vi "Autonomous Independent.vi"() -> ()   [LabVIEW 2019]
doc: "This VI is called when autonomous begins, and will automatically be terminated when autonomous ends. You can carry out timed or sensor driven robot movement independently without needing to return to the caller."
uses:
  <vilib>/Rock Robotics/Network Tables/NT Read String.vi
  Refnums.vi
  <vilib>/Rock Robotics/WPI/ThirdParty/Phoenix-LabVIEW/Motor Controller/Get/CTRE_Phoenix_MotorController_GetQuadratureData.vi
  <vilib>/addons/control/pid/pid.llb/PID (DBL).vi
  <vilib>/Rock Robotics/WPI/RobotDrive/WPI_RobotDriveArcadeDrive_Standard(NoSaturation).vi
  <vilib>/addons/control/pid/NI_PID_pid.lvlib
  <vilib>/Rock Robotics/WPI/ThirdParty/Phoenix-LabVIEW/Motor Controller/Controls/CTRE_Phoenix_MotorControl_ControlMode.ctl
panel:
  in  "Autonomous Step":T1(array[cluster]) {"Speed" min=0.0 max=1.0 step=0.01}
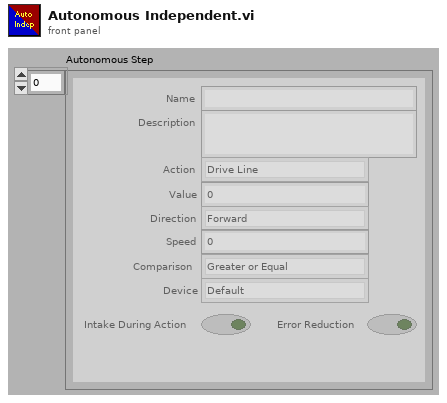
[diagram p1: front panel]
types:
  T1 = cluster{"Name":string, "Description":string, "Action":enum16{"Drive Line", "Drive Turn", "Drive Stop", "Drive Wait", "Shoot", ""}, "Value":dbl, "Direction":enum16{"Forward", "Reverse", "Left", "Right"}, "Speed":dbl, "Comparison":enum16{"Greater or Equal", "Less or Equal", "No compare (fixed)"}, "Device":enum16{"Default", "Gyro", "Laser", "Lidar", "Lime Light", "Encoder"}, "Intake During Action":bool, "Error Reduction":bool}[]
  T2 = typedef "WPI_RobotDriveDevRef.ctl" = cluster{"DevStatus":errorcluster, "Motors[]":T3[], "Square Inputs":bool, "Max Output":dbl}
  T3 = typedef "WPI_MotorControlDeviceRef.ctl" = cluster{"DeviceStatus":errorcluster, "Type":T4, "PWM":cluster{"PWM Channel":T5, "DeadBand":T6}, "CAN":cluster{"Device Number":u8, "SetOutput VI Ref":variant, "GetOutput VI Ref":variant, "Enable VI Ref":variant, "Disable VI Ref":variant, "Data":variant}, "Invert":bool, "DIO PWM":cluster{"PWM \"Enable\" Channel":T5, "DIOChannel":T7, "PWM Rate":dbl}}
  T4 = typedef "WPI_MotorControlType.ctl" = enum16{"PWM", "CAN", "DIO PWM"}
  T5 = typedef "FPGA_DIOPWMChannel.ctl" = enum8{"PWM 0", "PWM 1", "PWM 2", "PWM 3", "PWM 4", "PWM 5", "PWM 6", "PWM 7", "PWM 8", "PWM 9", "PWM MXP 0", "PWM MXP 1", "PWM MXP 2", "PWM MXP 3", "PWM MXP 4", "PWM MXP 5", "PWM MXP 6", "PWM MXP 7", "PWM MXP 8", "PWM MXP 9", "Invalid"}
  T6 = typedef "WPI_PWMDeadband.ctl" = cluster{"Name":string, "maxPositivePwm":i32, "minPositivePwm":i32, "centerPwm":i32, "maxNegativePwm":i32, "minNegativePwm":i32, "angularRange":u16}
  T7 = typedef "FPGA_DIOChannel.ctl" = enum8{"DIO 0", "DIO 1", "DIO 2", "DIO 3", "DIO 4", "DIO 5", "DIO 6", "DIO 7", "DIO 8", "DIO 9", "DIO MXP 0", "DIO MXP 1", "DIO MXP 2", "DIO MXP 3", "DIO MXP 4", "DIO MXP 5", "DIO MXP 6", "DIO MXP 7", "DIO MXP 8", "DIO MXP 9", "DIO MXP 10", "DIO MXP 11", "DIO MXP 12", "DIO MXP 13", "DIO MXP 14", "DIO MXP 15", "SPI Port CS1", "SPI Port CS2", "SPI Port CS3", "SPI Port MISO", "SPI Port MOSI", "Invalid"}
  T8 = cluster{"ROBOT_DRIVE":T2, "SHOOTER":T3, "RIGHT_DRIVE":T3, "LEFT_DRIVE":T3, "TURRET":T3, "SHOOTER SLAVE":T3, "INTAKE PIVOT":T3}
  T9 = cluster{"proportional gain (Kc)":dbl, "integral time (Ti, min)":dbl, "derivative time (Td, min)":dbl}
  T10 = enum16{"Drive Line", "Drive Turn", "Drive Stop", "Drive Wait", "Shoot", ""}
  T11 = enum16{"Greater or Equal", "Less or Equal", "No compare (fixed)"}
  T12 = enum16{"Default", "Gyro", "Laser", "Lidar", "Lime Light", "Encoder"}
  T13 = typedef "CTRE_Phoenix_MotorControl_ControlMode.ctl" = u16
  T14 = cluster{"Yaw":dbl, "Roll":dbl, "Pitch":dbl, "Heading":dbl, "Fused Heading":dbl}
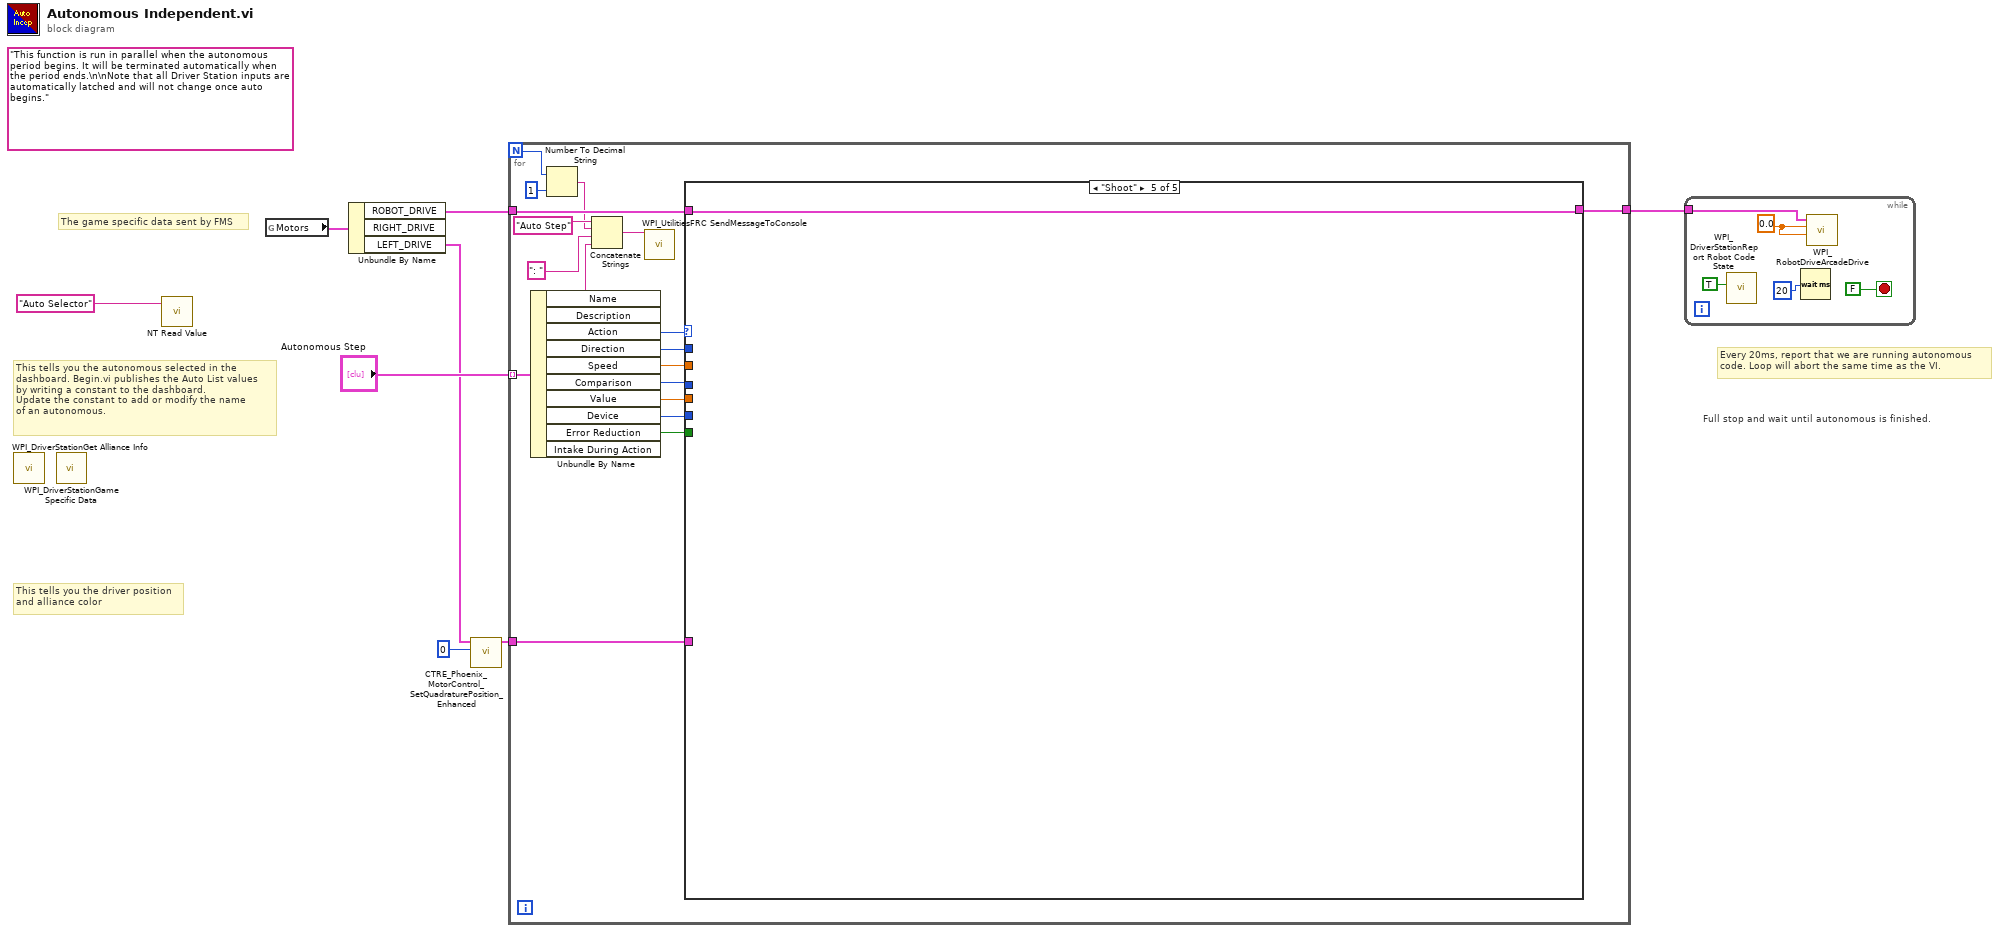
[diagram p0: block diagram]
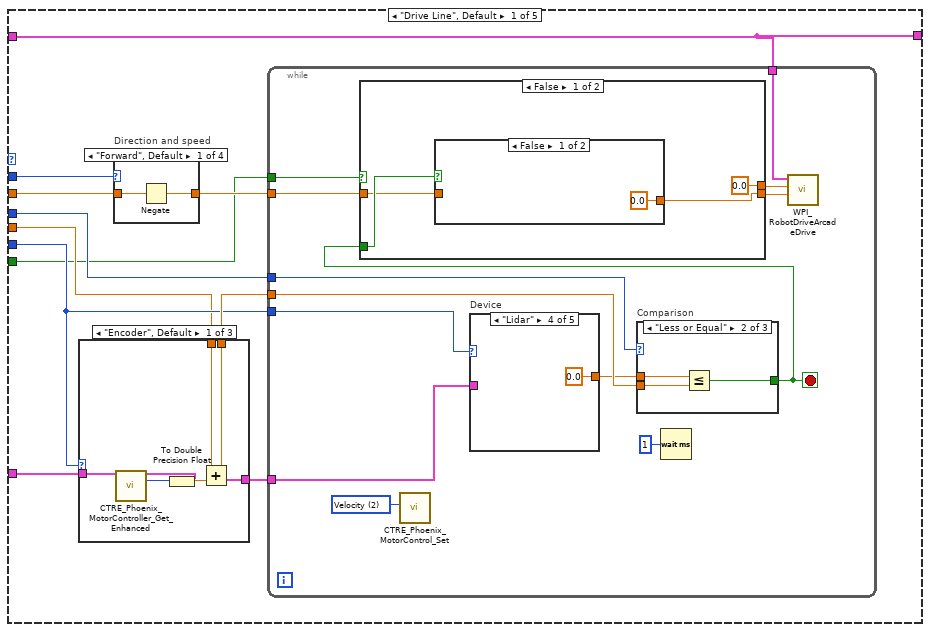
[diagram p2: hidden frame]
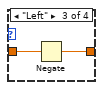
[diagram p6: hidden frame]
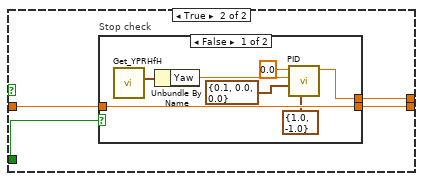
[diagram p9: hidden frame]
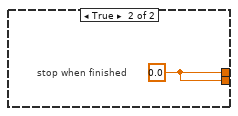
[diagram p10: hidden frame]
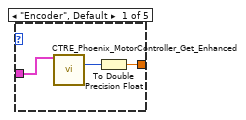
[diagram p11: hidden frame]
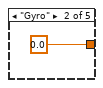
[diagram p12: hidden frame]
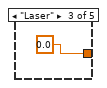
[diagram p13: hidden frame]
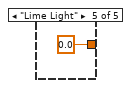
[diagram p14: hidden frame]
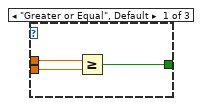
[diagram p15: hidden frame]
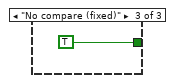
[diagram p16: hidden frame]
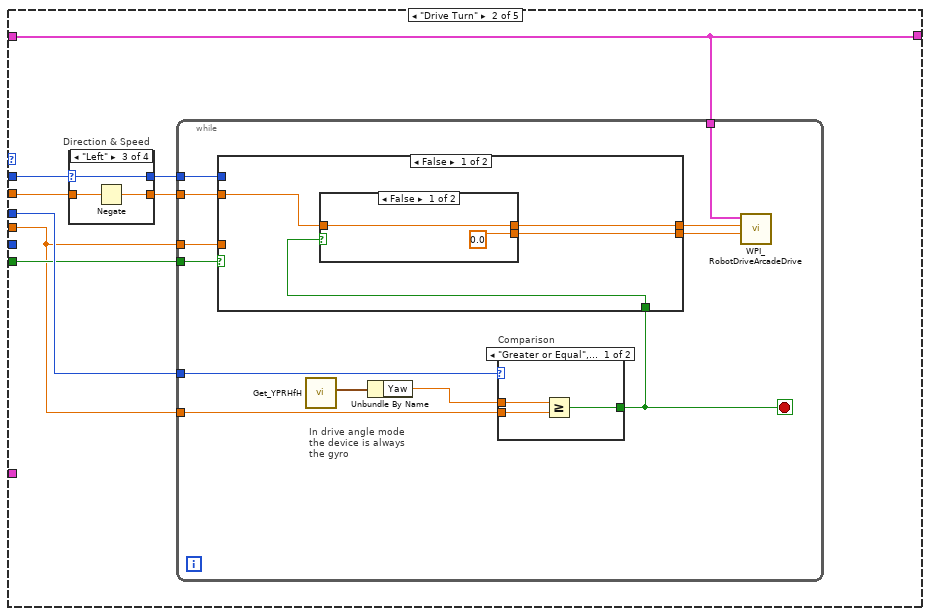
[diagram p17: hidden frame]
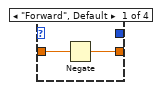
[diagram p18: hidden frame]
diagram:
  (unwired) "This function is run in parallel when the autonomous period begins. It will be terminated automatically when the period ends.\n\nNote that all Driver Station inputs are automatically latched and will not change once auto begins."
  # "Full stop and wait until autonomous is finished."
  # "The game specific data sent by FMS"
  # "This tells you the autonomous selected in the \ndashboard. Begin.vi publishes the Auto List values\nby writing a constant to the dashboard.\nUpdate the constant to add or modify the name\nof an autonomous."
  # "Every 20ms, report that we are running autonomous\ncode. Loop will abort the same time as the VI."
  # "This tells you the driver position\nand alliance color"
  n1 = call <vilib>:"WPI_DriverStationGet Alliance Info.vi"() -> ()  [unwired: 12 out]
  n2 = call <vilib>:"WPI_DriverStationGame Specific Data.vi"() -> ()  [unwired: 11 in, 1 out]
  n3 = call-poly <vilib>:"NT Read Value.vi"("Name"="Auto Selector") -> ()  [unwired: 9 in, 2 out]
  n4 = global read "Refnums.vi" "Motors"() -> (w6:T8)
  n5 = Unbundle By Name(w6) -> ("ROBOT_DRIVE"=w3:T2, "LEFT_DRIVE"=w1:T3)  [unwired: 1 out]
  n6 = call <vilib>:"CTRE_Phoenix_MotorControl_SetQuadraturePosition_Enhanced.vi"("New Position"=0, "PhoenixMotorControlDevRef"=w1) -> ("PhoenixMotorControlDevRef"=w4:T3)  [unwired: 8 in, 1 out]
  n7 = for {
    N -> [w11]
    tunnel: "Autonomous Step" -> [w26] mode=indexing
    tunnel: w4 -> [w18]
    tunnel: w3 -> [w17]
    tunnel: [w16] -> w2
    n8 = Unbundle By Name(w26) -> ("Name"=w14:string, "Action"=w25:T10, "Direction"=w24:enum16{"Forward", "Reverse", "Left", "Right"}, "Speed"=w23:dbl, "Comparison"=w19:T11, "Value"=w20:dbl, "Device"=w22:T12, "Error Reduction"=w21:bool)  [unwired: 2 out]
    n9 = Number To Decimal String(number=w11, width (-)=i16 1) -> (decimal integer string=w9:string)
    n10 = Concatenate Strings("Auto Step" ("string"), w9, ": " ("string"), w14) -> (w15:string)
    n11 = call <vilib>:"WPI_UtilitiesFRC SendMessageToConsole.vi"("Message"=w15) -> ()  [unwired: 14 in, 1 out]
    n12 = case shown="\"Shoot\"" w25 {
      tunnel: w24 -> [w32 w103 _ _ _]
      tunnel: w23 -> [w33 w105 _ _ _]
      tunnel: w22 -> [w34 _ _ _ _]
      tunnel: w21 -> [w27 w101 _ _ _]
      tunnel: w20 -> [w31 w99 _ w162 _]
      tunnel: w19 -> [w30 w104 _ _ _]
      tunnel: w18 -> [w29 _ _ _ _]
      tunnel: w17 -> [w28 w102 w160 w163 w164]
      tunnel: [w28 w102 w160 w163 w164] -> w16
      frame "Drive Line", Default {
        n13 = case shown="\"Encoder\", Default" w34 {
          tunnel: w29 -> [w43 w44 w46]
          tunnel: w31 -> [w40 w45 w47]
          tunnel: [w39 w45 w47] -> w36
          tunnel: [w38 w44 w46] -> w35
          frame "Encoder", Default {
            n14 = call-poly <vilib>:"CTRE_Phoenix_MotorController_Get_Enhanced.vi"("PhoenixMotorControlDevRef"=w43) -> ("PhoenixMotorControlDevRef"=w38:T3, "Quadrature Position"=w41:i32)  [unwired: 11 in, 2 out]
            n15 = To Double Precision Float(number=w41) -> (double precision float=w42:dbl)
            n16 = Add(x=w40, y=w42) -> (x+y=w39:dbl)
          }
          frame "Gyro" {
          }
          frame "Laser" {
          }
        }
        n17 = case "Direction and speed" shown="\"Forward\", Default" w32 {
          tunnel: w33 -> [w48 w50 w51 w53]
          tunnel: [w49 w50 w52 w53] -> w37
          frame "Forward", Default {
            n18 = Negate(x=w48) -> (-x=w49:dbl)
          }
          frame "Reverse" {
          }
          frame "Left" {
            n19 = Negate(x=w51) -> (-x=w52:dbl)
          }
          frame "Right" {
          }
        }
        n20 = while {
          tunnel: w30 -> [w61]
          tunnel: w36 -> [w66]
          tunnel: w37 -> [w65]
          tunnel: w34 -> [w60]
          tunnel: w28 -> [w62]
          tunnel: w35 -> [w58]
          tunnel: w27 -> [w54]
          stop <- w56 stop-if-true
          w55 = T13 2 items=["PercentOutput"=0, "Position"=1, "Velocity"=2, "Current"=3, "Follower"=5, "MotionProfile"=6, "MotionMagic"=7, "MotionProfileArc"=10, "Disabled"=15] ("Control Mode")
          n21 = call <vilib>:"CTRE_Phoenix_MotorControl_Set.vi"("Control Mode"=w55) -> ()  [unwired: 9 in, 2 out]
          n22 = case "Device" shown="\"Lidar\"" w60 {
            tunnel: [w86 0.0 0.0 0.0 0.0] -> w59
            tunnel: w58 -> [w87 _ _ _ _]
            frame "Encoder", Default {
              n23 = call-poly <vilib>:"CTRE_Phoenix_MotorController_Get_Enhanced.vi"("PhoenixMotorControlDevRef"=w87) -> ("Quadrature Position"=w85:i32)  [unwired: 11 in, 3 out]
              n24 = To Double Precision Float(number=w85) -> (double precision float=w86:dbl)
            }
            frame "Gyro" {
            }
            frame "Laser" {
            }
            frame "Lidar" {
            }
            frame "Lime Light" {
            }
          }
          n25 = case "Comparison" shown="\"Less or Equal\"" w61 {
            tunnel: [w94 w97 TRUE] -> w56
            tunnel: w66 -> [w93 w96 _]
            tunnel: w59 -> [w92 w95 _]
            frame "Greater or Equal", Default {
              n26 = Greater Or Equal?(x=w92, y=w93) -> (x >= y?=w94:bool)
            }
            frame "Less or Equal" {
              n27 = Less Or Equal?(x=w95, y=w96) -> (x <= y?=w97:bool)
            }
            frame "No compare (fixed)" {
            }
          }
          n28 = case shown="False" w54 {
            tunnel: w65 -> [w68 w76]
            tunnel: [0.0 ("X axis value") w75] -> w64
            tunnel: [w67 w74] -> w63
            tunnel: w56 -> [w69 w73]
            frame False {
              n29 = case shown="False" w69 {
                tunnel: w68 -> [_ w72]
                tunnel: [0.0 ("Speed") w72] -> w67
                frame False {
                }
                frame True {
                }
              }
            }
            frame True {
              n30 = case "Stop check" shown="False" w73 {
                tunnel: w76 -> [w83 _]
                tunnel: [w82 w84] -> w75
                tunnel: [w83 w84] -> w74
                frame False {
                  n31 = call <vilib>:"Get_YPRHfH.vi"() -> ("YRPHfH"=w78:T14)  [unwired: 11 in]
                  n32 = Unbundle By Name(w78) -> ("Yaw"=w77:dbl)
                  n33 = call-poly <vilib>:"PID.vi"("output range"=cluster{"output high":dbl, "output low":dbl} {"output high"=1.0, "output low"=-1.0}, "PID gains"=T9 {"proportional gain (Kc)"=0.1, "integral time (Ti, min)"=0.0, "derivative time (Td, min)"=0.0}, "process variable"=w77, "setpoint"=0.0) -> ("output"=w82:dbl)  [unwired: 6 in, 1 out]
                }
                frame True {
                  w84 = 0.0 ("X axis value")
                  # "stop when finished"
                }
              }
            }
          }
          n34 = Wait (ms)(milliseconds to wait=u32 1) -> ()  [unwired: 1 out]
          n35 = call-poly <vilib>:"WPI_RobotDriveArcadeDrive.vi"("Y axis value"=w63, "X axis value"=w64, "RobotDriveDevRef"=w62) -> ()  [unwired: 1 in, 8 out]
        }
      }
      frame "Drive Turn" {
        n36 = case "Direction & Speed" shown="\"Left\"" w103 {
          selector: w103 -> [_ _ w110 _]
          tunnel: w105 -> [w107 w109 w111 w113]
          tunnel: [w108 w109 w112 w113] -> w106
          tunnel: [_ _ w110 _] -> w100
          frame "Forward", Default {
            n37 = Negate(x=w107) -> (-x=w108:dbl)
          }
          frame "Reverse" {
          }
          frame "Left" {
            n38 = Negate(x=w111) -> (-x=w112:dbl)
          }
          frame "Right" {
          }
        }
        n39 = while {
          tunnel: w104 -> [w118]
          tunnel: w99 -> [w117]
          tunnel: w106 -> [w125]
          tunnel: w102 -> [w122]
          tunnel: w101 -> [w121]
          tunnel: w100 -> [w116]
          tunnel: w99 -> [w115]
          stop <- w114 stop-if-true
          # "In drive angle mode\nthe device is always\nthe gyro"
          n40 = call <vilib>:"Get_YPRHfH.vi"() -> ("YRPHfH"=w119:T14)  [unwired: 11 in]
          n41 = Unbundle By Name(w119) -> ("Yaw"=w120:dbl)
          n42 = case "Comparison" shown="\"Greater or Equal\", Default" w118 {
            tunnel: [w128 w131] -> w114
            tunnel: w120 -> [w127 w130]
            tunnel: w117 -> [w126 w129]
            frame "Greater or Equal", Default {
              n43 = Greater Or Equal?(x=w127, y=w126) -> (x >= y?=w128:bool)
            }
            frame "Less or Equal" {
              n44 = Less Or Equal?(x=w130, y=w129) -> (x <= y?=w131:bool)
            }
          }
          n45 = case shown="False" w121 {
            tunnel: w125 -> [w135 w147]
            tunnel: [w134 w142] -> w124
            tunnel: [w133 0.0 ("X axis value")] -> w123
            tunnel: w116 -> [_ w140]
            tunnel: w115 -> [_ w139]
            tunnel: w114 -> [w132 _]
            frame False {
              n46 = case shown="False" w132 {
                tunnel: w135 -> [w137 _]
                tunnel: [w137 w138] -> w134
                tunnel: [0.0 ("X axis value") w138] -> w133
                frame False {
                }
                frame True {
                  w138 = 0.0 ("X axis value")
                }
              }
            }
            frame True {
              n47 = case shown="\"Forward\"" w140 {
                tunnel: w147 -> [w148 w153 w155 w159]
                tunnel: [w150 w151 w154 w157] -> w146
                frame "Reverse" {
                  n48 = Bundle("Speed"=w148, 0.0) -> (w150:cluster{"Speed":dbl, dbl})  [unwired: 1 in]
                }
                frame "Forward" {
                  n49 = Bundle(0.0, "Speed"=w153) -> (w151:cluster{dbl, "Speed":dbl})  [unwired: 1 in]
                }
                frame "Right", Default {
                  n50 = Bundle("Speed"=w155, 0.0) -> (w154:cluster{"Speed":dbl, dbl})  [unwired: 1 in]
                }
                frame "Left" {
                  n51 = Bundle(0.0, "Speed"=w159) -> (w157:cluster{dbl, "Speed":dbl})  [unwired: 1 in]
                }
              }
              n52 = call <vilib>:"Get_YPRHfH.vi"() -> ("YRPHfH"=w145:T14)  [unwired: 11 in]
              n53 = Unbundle By Name(w145) -> ("Yaw"=w144:dbl)
              n54 = global read "PID.vi" "TURNING"() -> (w143:cluster{"P":dbl, "I":dbl, "D":dbl})
              n55 = call-poly <vilib>:"PID.vi"("output range"=w146, "PID gains"=w143, "process variable"=w144, "setpoint"=w139) -> ("output"=w142:dbl)  [unwired: 6 in, 1 out]
            }
          }
          n56 = call-poly <vilib>:"WPI_RobotDriveArcadeDrive.vi"("Y axis value"=w123, "X axis value"=w124, "RobotDriveDevRef"=w122) -> ()  [unwired: 1 in, 8 out]
        }
      }
      frame "Drive Stop" {
        w161 = 0.0 ("X axis value")
        # "Stop all drive motion"
        n57 = call-poly <vilib>:"WPI_RobotDriveArcadeDrive.vi"("Y axis value"=w161, "X axis value"=w161, "RobotDriveDevRef"=w160) -> ()  [unwired: 1 in, 8 out]
      }
      frame "Drive Wait" {
        n58 = call <vilib>:"WPI_RobotDriveDelayAndUpdateSafety.vi"("Delay (s)"=w162, "RobotDriveDevRef"=w163) -> ()  [unwired: 8 in, 2 out]
      }
      frame "Shoot" {
      }
    }
  }
  n59 = while {
    tunnel: w2 -> [w166]
    stop <- FALSE stop-if-true
    w165 = 0.0 ("X axis value")
    n60 = call <vilib>:"WPI_DriverStationReport Robot Code State.vi"("Autonomous"=TRUE) -> ()  [unwired: 10 in, 1 out]
    n61 = Wait (ms)(milliseconds to wait=u32 20) -> ()  [unwired: 1 out]
    n62 = call-poly <vilib>:"WPI_RobotDriveArcadeDrive.vi"("Y axis value"=w165, "X axis value"=w165, "RobotDriveDevRef"=w166) -> ()  [unwired: 6 in, 3 out]
  }
